vi "save.vi"(5 "log?":bool, 8 "queue in":refnum<queue>, 11 "Qube":refnum<class "System.lvclass">) -> (3 "Qube":refnum<class "System.lvclass">)   [LabVIEW 2021, in "System.lvclass"]
uses:
  System.lvclass
  System.lvclass/System.ctl
panel:
  out "error out":errorcluster
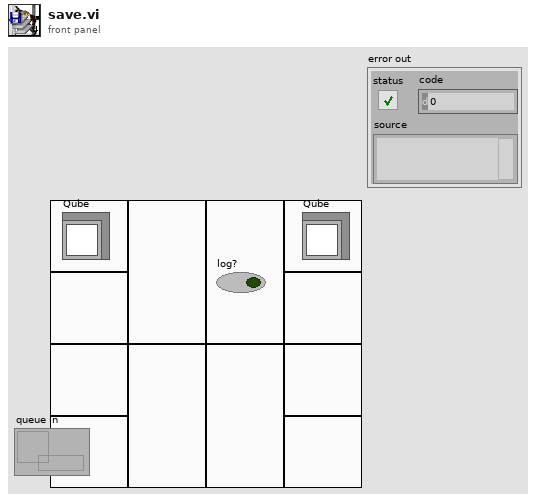
[diagram p1: front panel]
types:
  T1 = enum16{"big-endian, network order", "native, host order", "little-endian"}
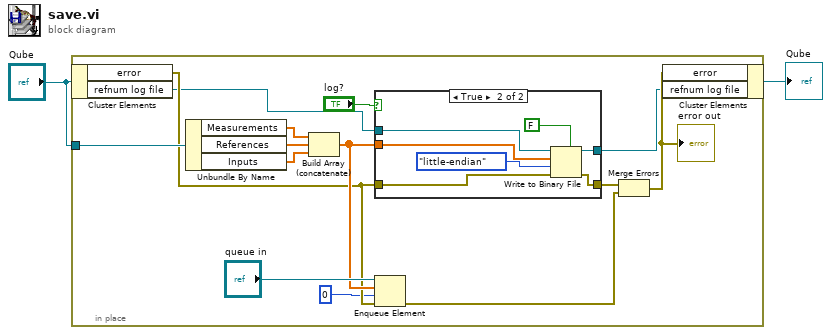
[diagram p0: block diagram]
diagram:
  n1 = in-place {
    in-place-border: "Qube" -> [w16]
    n2 = in-place-cluster #1("Qube") -> ("error"=w6:errorcluster, "refnum log file"=w5:refnum<file>)
    n3 = Unbundle By Name(w16) -> ("Measurements"=w15:dbl[], "References"=w14:dbl[], "Inputs"=w13:dbl[])
    n4 = Build Array (concatenate)(w15, w14, w13) -> (w10:dbl[])
    n5 = case shown="True" "log?" {
      tunnel: w6 -> [w17 w24]
      tunnel: w10 -> [_ w22]
      tunnel: w5 -> [w18 w21]
      tunnel: [w17 w20] -> w8
      tunnel: [w18 w19] -> w4
      frame False {
      }
      frame True {
        n6 = Write to Binary File(file (use dialog)=w21, data=w22, error in=w24, 5:FALSE ("prepend array or string size? (T)"), 9:T1."little-endian" ("byte order (0:big-endian, network order)")) -> (refnum out=w19:refnum<file>, error out=w20:errorcluster)  [unwired: 1 in, 1 out]
      }
    }
    n7 = Enqueue Element(queue="queue in", element=w10, timeout in ms (-1)=0, error in (no error)=w6) -> (error out=w9:errorcluster)  [unwired: 2 out]
    n8 = Merge Errors(w8, w9) -> (w7:errorcluster)
    "error out" <- w7
    n9 = in-place-cluster #1("error"=w7, "refnum log file"=w4) -> (→"Qube":refnum<class "System.lvclass">)
  }
